vi "PixieDAQControlState.vi"() -> ()   [LabVIEW 2011]
panel:
  in  "ContDAQ":bool
  in  "Run Parameters":T1={"Block time (s)"=1.0, "Max Runtime (s)"=10.0, "Max Counts"=10000, "C12 Limit"=0.0, "Max BadBlocks"=100} {"Block time (s)" min=0.0 max=100.0 step=0.1}
  in  "StartDAQ":bool
  out "Run Data":T2={"C12"=1.1914090738075305, "C13L"=0.5017245101686503, "C13H"=0.5034155301731089, "Counts"=367, "LT"=6.561814399999999, "RT"=6.564085759999999, "BadBlocks"=0, "C1312"=0.0}
  out "Run Ratios":T3 {"DTfrac" format="%#_3f"}
  out "Acquiring":bool
  in  "stop":bool
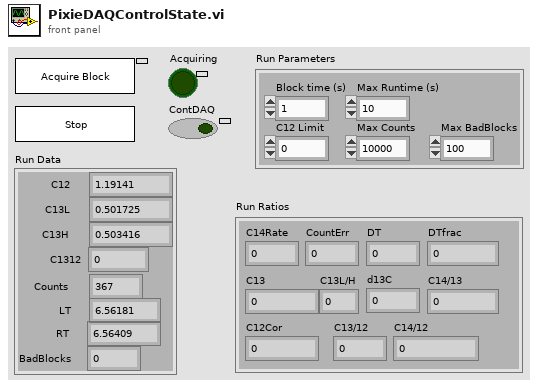
[diagram p1: front panel]
types:
  T1 = cluster{"Block time (s)":dbl, "Max Runtime (s)":dbl, "Max Counts":u32, "C12 Limit":dbl, "Max BadBlocks":u8}
  T2 = cluster{"C12":dbl, "C13L":dbl, "C13H":dbl, "Counts":u32, "LT":dbl, "RT":dbl, "BadBlocks":u8, "C1312":dbl}
  T3 = cluster{"C14Rate":dbl, "CountErr":dbl, "DT":dbl, "DTfrac":dbl, "C13":dbl, "C13L/H":dbl, "d13C":dbl, "C14/13":dbl, "C12Cor":dbl, "C13/12":dbl, "C14/12":dbl}
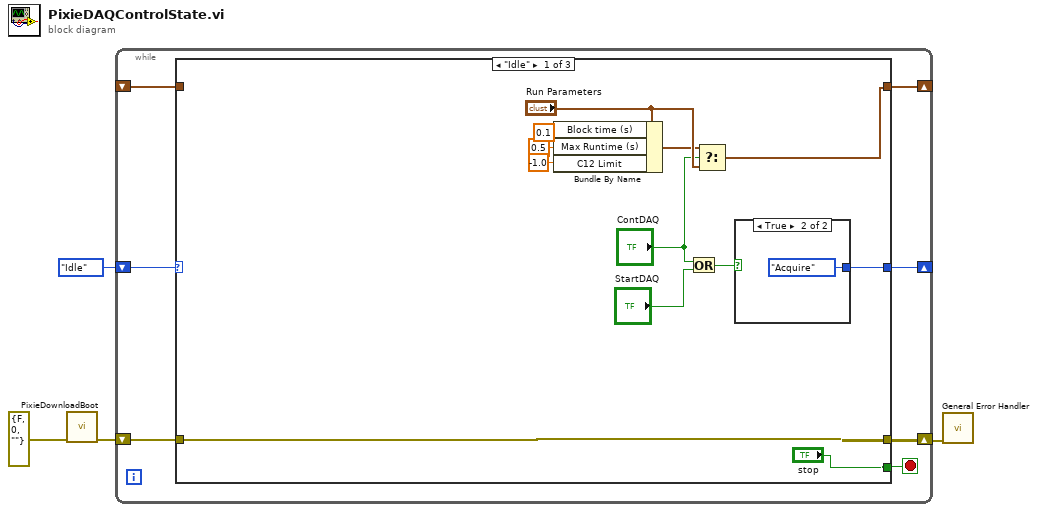
[diagram p0: block diagram]
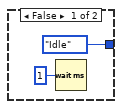
[diagram p2: hidden frame]
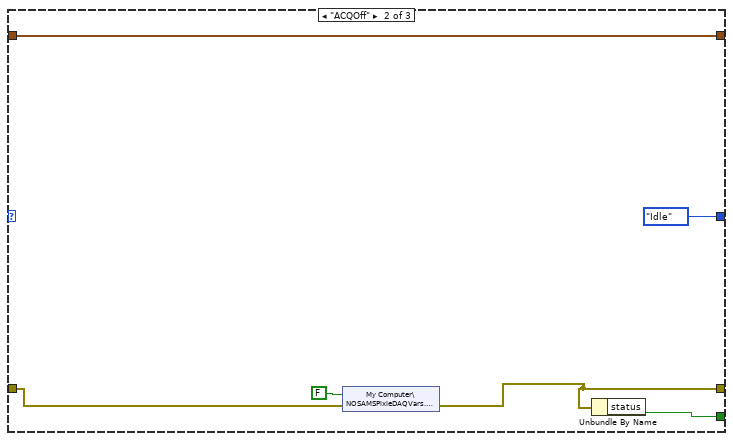
[diagram p3: hidden frame]
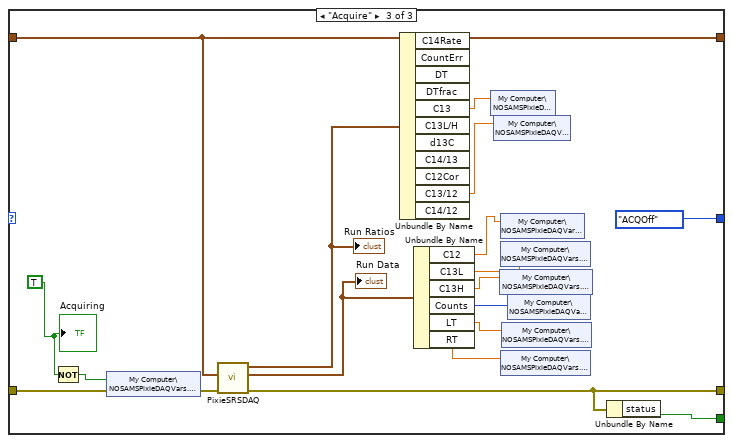
[diagram p4: hidden frame]
diagram:
  n1 = call "PixieDownloadBoot.vi"("error in (no error)"=errorcluster {"status"=FALSE, "code"=0, "source"=""} ("error IO")) -> ("error out"=w2:errorcluster)  [unwired: 5 in, 5 out]
  n2 = while {
    shift-right: [w10] -> w4
    shift-left: w2 -> [w9]
    shift-right: [w7] -> _
    shift-left: enum16{"Idle", "Acquire", "ACQOff"}."Idle" -> [w8]
    shift-right: [w5] -> _
    shift-left: _ -> [w6]
    stop <- w11 stop-if-true
    n3 = case shown="\"Idle\"" w8 {
      tunnel: ["stop" w29 w38] -> w11
      tunnel: [w22 w30 w37] -> w10
      tunnel: w9 -> [w22 w31 w50]
      tunnel: [w21 enum16{"Idle", "Acquire", "ACQOff"}."Idle" enum16{"Idle", "Acquire", "ACQOff"}."ACQOff"] -> w7
      tunnel: w6 -> [_ w27 w34]
      tunnel: [w12 w27 w34] -> w5
      frame "Idle" {
        n4 = Bundle By Name(cluster="Run Parameters", "Block time (s)"=0.1, "Max Runtime (s)"=0.5, "C12 Limit"=-1.0) -> (w17:T1)
        n5 = Or(x="ContDAQ", y="StartDAQ") -> (x .or. y?=w19:bool)
        n6 = Select(t=w17, s="ContDAQ", f="Run Parameters") -> (s? t:f=w12:T1)
        n7 = case shown="True" w19 {
          tunnel: [enum16{"Idle", "Acquire", "ACQOff"}."Idle" enum16{"Idle", "Acquire", "ACQOff"}."Acquire"] -> w21
          frame False {
            n8 = Wait (ms)(milliseconds to wait=u32 1) -> ()  [unwired: 1 out]
          }
          frame True {
          }
        }
      }
      frame "ACQOff" {
        n9 = shared-variable "My Computer\\NOSAMSPixieDAQVars.lvlib\\Acquiring"(FALSE ("Acquire"), error in=w31) -> (error out=w30:errorcluster)
        n10 = Unbundle By Name(w30) -> ("status"=w29:bool)
      }
      frame "Acquire" {
        w33 = TRUE
        n11 = Not(x=w33) -> (.not. x?=w35:bool)
        n12 = shared-variable "My Computer\\NOSAMSPixieDAQVars.lvlib\\StartDAQ"(w35, error in=w50) -> (error out=w49:errorcluster)
        n13 = call "PixieSRSDAQ.vi"("error in (no error)"=w49, "Run Parameters"=w34) -> ("error out"=w37:errorcluster, "Run Data"=w48:T2, "Run Ratios"=w41:T3)  [unwired: 7 out]
        "Run Ratios" <- w41
        "Run Data" <- w48
        n14 = Unbundle By Name(w41) -> ("C13"=w39:dbl, "C13/12"=w40:dbl)  [unwired: 9 out]
        n15 = Unbundle By Name(w48) -> ("C12"=w47:dbl, "C13L"=w46:dbl, "C13H"=w45:dbl, "Counts"=w44:u32, "LT"=w43:dbl, "RT"=w42:dbl)
        n16 = shared-variable "My Computer\\NOSAMSPixieDAQVars.lvlib\\C13"(w39) -> ()  [unwired: 2 out]
        n17 = shared-variable "My Computer\\NOSAMSPixieDAQVars.lvlib\\C1312"(w40) -> ()  [unwired: 2 out]
        n18 = shared-variable "My Computer\\NOSAMSPixieDAQVars.lvlib\\C13HCur"(w45) -> ()  [unwired: 2 out]
        n19 = shared-variable "My Computer\\NOSAMSPixieDAQVars.lvlib\\C12Cur"(w47) -> ()  [unwired: 2 out]
        n20 = shared-variable "My Computer\\NOSAMSPixieDAQVars.lvlib\\C13LCur"(w46) -> ()  [unwired: 2 out]
        n21 = shared-variable "My Computer\\NOSAMSPixieDAQVars.lvlib\\Runtime"(w42) -> ()  [unwired: 2 out]
        n22 = shared-variable "My Computer\\NOSAMSPixieDAQVars.lvlib\\Livetime"(w43) -> ()  [unwired: 2 out]
        n23 = shared-variable "My Computer\\NOSAMSPixieDAQVars.lvlib\\Counts"(w44) -> ()  [unwired: 2 out]
        n24 = Unbundle By Name(w37) -> ("status"=w38:bool)
        "Acquiring" <- w33
      }
    }
  }
  n25 = call <vilib>:"General Error Handler.vi"("error in (no error)"=w4) -> ()  [unwired: 1 in, 14 out]
